vi "_061.vi"() -> ()   [LabVIEW 2024]
uses:
  <vilib>/measure/NI_MABase.lvlib
panel:
  in  "signal type":T1(ring)
  out "Waveform Graph":waveform(dbl)(graph)
  in  "amplitude":dbl(knob)=1.0 scale=0.0..10.0
  in  "frequency":dbl(knob)=10.0 scale=0.0..10.0
  # "To write the live data :"
  # "( Using Write to Measurement File )"
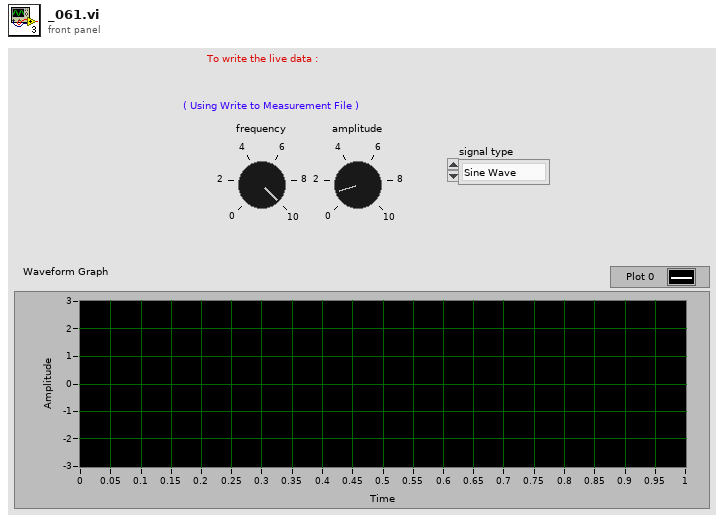
[diagram p1: front panel]
types:
  T1 = enum16{"Sine Wave", "Triangle Wave", "Square Wave", "Sawtooth Wave"}
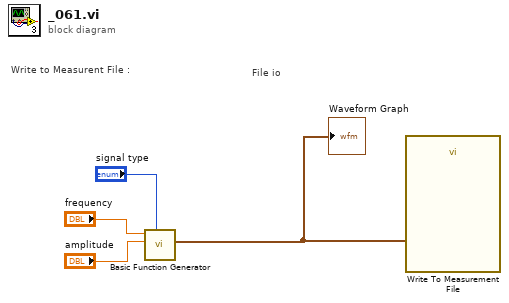
[diagram p0: block diagram]
diagram:
  # "File io"
  # "Write to Measurent File :"
  n1 = call <vilib>:"Basic Function Generator.vi"("signal type"="signal type", "amplitude"="amplitude", "frequency"="frequency") -> ("signal out"=w2:waveform(dbl))  [unwired: 6 in, 2 out]
  "Waveform Graph" <- w2
  n2 = call "Write To Measurement File"("Signals"=w2) -> ()  [unwired: 16 in, 3 out]
